vi "Initialize Diagnostics File.vi"() -> (0 "error out":errorcluster, 3 "diagnostics file":refnum<file>)   [LabVIEW 2021, in "Diagnostics.lvlib"]
doc: "Initialize the debug log file."
uses:
  Diagnostics.lvlib
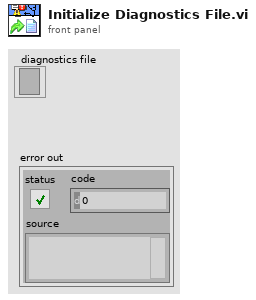
[diagram p1: front panel]
types:
  T1 = enum16{"open", "replace", "create", "open or create", "replace or create", "replace or create with confirmation"}
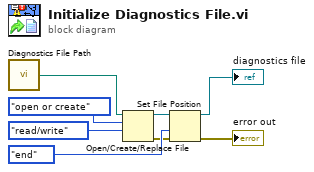
[diagram p0: block diagram]
diagram:
  n1 = call "Diagnostics File Path.vi"() -> ("diagnostics file path"=w3:path)
  n2 = Open/Create/Replace File(file path (use dialog)=w3, operation (0:open)=T1."open or create", access (0:read/write)=enum16{"read/write", "read-only", "write-only"}."read/write") -> (refnum out=w5:refnum<file>, error out=w4:errorcluster)  [unwired: 3 in, 1 out]
  n3 = Set File Position(refnum=w5, from (0:start)=enum16{"start", "end", "current"}."end", error in=w4) -> (refnum out=→"diagnostics file":refnum<file>, error out=→"error out":errorcluster)  [unwired: 1 in]
